vi "ESC Control v1.vi"() -> ()   [LabVIEW 2016]
uses:
  <vilib>/MakerHub/LINX/Public/Utilities/Open Serial.vi
  <vilib>/MakerHub/LINX/Public/Sensors/Motion/Servo/Servo Open One Channel.vi
  <vilib>/MakerHub/LINX/Public/Sensors/Motion/Servo/Servo Set Pulse Width One Channel.vi
  <vilib>/MakerHub/LINX/Public/Sensors/Motion/Servo/Servo Close One Channel.vi
  <vilib>/MakerHub/LINX/LMH-LINX.lvlib
  <vilib>/MakerHub/LINX/Public/Sensors/Motion/Servo/Servo.lvlib
panel:
  out "Power % Gauge":dbl(knob) scale=0.0..100.0
  in  "Power %":dbl min=0.0 max=100.0 step=0.5 format="%.1f"
  in  "Stop Button":bool
  in  "Serial Port":refnum<visa-resource-name>
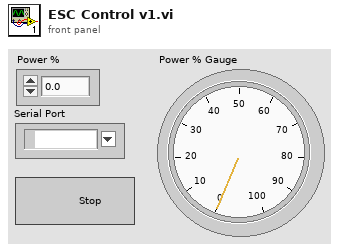
[diagram p1: front panel]
types:
  T1 = typedef "LMH-LINX.lvlib/LINX Ref.ctl" = cluster{"IO":T2, "Interface":T3, "LINX Device Config":T4}
  T2 = typedef "LMH-LINX.lvlib/Platform.ctl" = enum16{"Remote", "Local"}
  T3 = typedef "LMH-LINX.lvlib/Interface.ctl" = enum16{"Serial", "TCP"}
  T4 = typedef "LMH-LINX.lvlib/Device.lvlib/LINX Device Config.ctl" = cluster{"Interface":T3, "COM Port":refnum<visa-resource-name>, "TCP Configuration":T5, "Device Family":u8, "Device ID":u8, "Device Name":string, "TCP Ref":refnum<k5>, "Channels":T6}
  T5 = typedef "LMH-LINX.lvlib/Device.lvlib/TCP Config.ctl" = cluster{"IP Address":string, "Port":u16}
  T6 = typedef "LMH-LINX.lvlib/Channels.ctl" = cluster{"DI":u8[], "DO":u8[], "AI":u8[], "AO":u8[], "PWM":u8[], "QE":u8[], "UART":u8[], "I2C 2":u8[], "SPI":u8[], "CAN":u8[], "Servo":u8[], "AI Ref (V)":dbl, "AI Resolution (Bits)":u8, "AO Ref (V)":dbl, "AO Resolution (Bits)":u8}
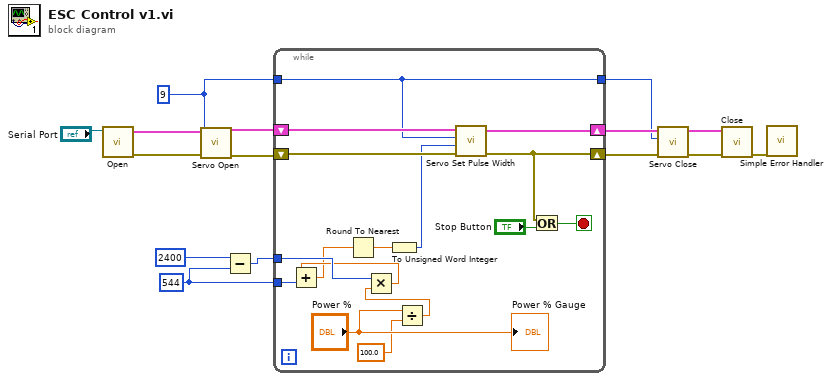
[diagram p0: block diagram]
diagram:
  w1 = 9
  w3 = 544
  n1 = call-poly <vilib>:"Open.vi"("Serial Port"="Serial Port") -> ("Error Out"=w14:errorcluster, "LINX Resource"=w13:T1)  [unwired: 8 in, 1 out]
  n2 = call-poly <vilib>:"Servo Open.vi"("Error In"=w14, "Servo Channel"=w1, "LINX Resource"=w13) -> ("Error Out"=w12:errorcluster, "LINX Resource"=w11:T1)  [unwired: 7 in]
  n3 = Subtract(x=2400, y=w3) -> (x-y=w2:i32)
  n4 = while {
    shift-right: [w28] -> w6
    shift-left: w12 -> [w29]
    tunnel: w1 -> [w25]
    shift-right: [w26] -> w9
    shift-left: w11 -> [w27]
    tunnel: [w25] -> w5
    tunnel: w3 -> [w22]
    tunnel: w2 -> [w21]
    stop <- w31 stop-if-true
    n5 = Divide(x="Power %", y=100.0) -> (x/y=w18:dbl)
    n6 = Multiply(x=w21, y=w18) -> (x*y=w17:dbl)
    n7 = Add(x=w17, y=w22) -> (x+y=w16:dbl)
    n8 = Round To Nearest(number=w16) -> (nearest integer value=w24:dbl)
    n9 = To Unsigned Word Integer(number=w24) -> (unsigned 16bit integer=w23:u16)
    n10 = call-poly <vilib>:"Servo Set Pulse Width.vi"("Error In"=w29, "Pulse Width (uS)"=w23, "Servo Channel"=w25, "LINX Resource"=w27) -> ("Error Out"=w28:errorcluster, "LINX Resource"=w26:T1)  [unwired: 6 in]
    n11 = Or(x=w28, y="Stop Button") -> (x .or. y?=w31:bool)
    "Power % Gauge" <- "Power %"
  }
  n12 = call-poly <vilib>:"Servo Close.vi"("Error In"=w6, "Servo Channel"=w5, "LINX Resource"=w9) -> ("Error Out"=w7:errorcluster, "LINX Resource"=w8:T1)  [unwired: 7 in]
  n13 = call <vilib>:"Close.vi"("Error In"=w7, "LINX Resource"=w8) -> ("Error Out"=w10:errorcluster)  [unwired: 9 in]
  n14 = call <vilib>:"Simple Error Handler.vi"("error in (no error)"=w10) -> ()  [unwired: 4 in, 5 out]
